vi "mod_Doppler Filter Taps.vi"(0 "doppler spread (hz)":dbl=0.001 format="%#_6p", 5 "fs":dbl=10.0, 7 "doppler filter length":i32=1000, 11 "error in (no error)":errorcluster, 13 "reset? (T)":bool=TRUE) -> (4 "doppler filter taps":dbl[](array[numeric]), 6 "doppler spectrum":dbl[](array[numeric]), 15 "error out":errorcluster)   [LabVIEW 2020, in "niDMT.lvlib"]
doc: "Design of a Doppler filter with U-shaped power spectral density in frequency domain.\n\n\n Inputs:\n 1) Doppler frequency (Hz) \n - range : double precision\n 2) sampling frequency : the sampling frequency of the input\n 3) number of frequency samples within Doppler frequency: the number of samples within the Doppler frequency in frequency domain, which mainly decides the resolution of the filter\n\n Outputs:\n 1) Doppler filter : the Doppler filter coefficient in frequency domain"
uses:
  <vilib>/addons/Modulation/niDMT.lvlib
  <vilib>/Analysis/2dsp.llb/Inverse Real FFT.vi
  <vilib>/Analysis/NI_AALPro.lvlib
panel:
  out "doppler spectrum":cluster{dbl, dbl, dbl[]}(graph)={-0.005, 0.0001, [0.0, 0.0, 0.0, 0.0, 0.0, 0.0, 0.0, 0.0, 0.0, 0.0, 0.0, 0.0, 0.0, 0.0, 0.0, 0.0, 0.0, 0.0, 0.0, 0.0, 0.0, 0.0, 0.0, 0.0, 0.0, 0.0, 0.0, 0.0, 0.0, 0.0, 0.0, 0.0, 0.0, 0.0, 0.0, 0.0, 0.0, 0.0, 0.0, 0.0, 3.3096517068365974, 2.8209479177387817, 2.5857000817159306, 2.4430125595146, 2.3480393851504964, 2.2824478932324883, 2.2372285100045572, 2.2075110436214076, 2.19059400363999, 2.1850968611841584, 2.1850968611841584, 2.19059400363999, 2.2075110436214076, 2.2372285100045572, 2.2824478932324883, 2.3480393851504964, 2.4430125595146, 2.5857000817159306, 2.8209479177387817, 3.3096517068365974, 0.0, 0.0, 0.0, 0.0, 0.0, 0.0, 0.0, 0.0, 0.0, 0.0, 0.0, 0.0, 0.0, 0.0, 0.0, 0.0, 0.0, 0.0, 0.0, 0.0, 0.0, 0.0, 0.0, 0.0, 0.0, 0.0, 0.0, 0.0, 0.0, 0.0, 0.0, 0.0, 0.0, 0.0, 0.0, 0.0, 0.0, 0.0, 0.0, 0.0]}
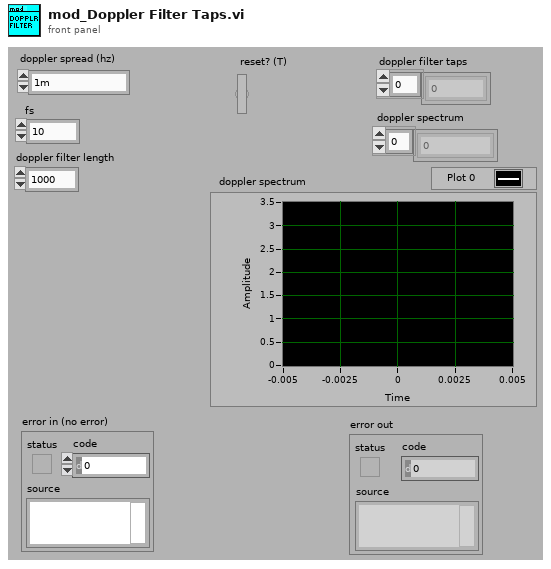
[diagram p1: front panel]
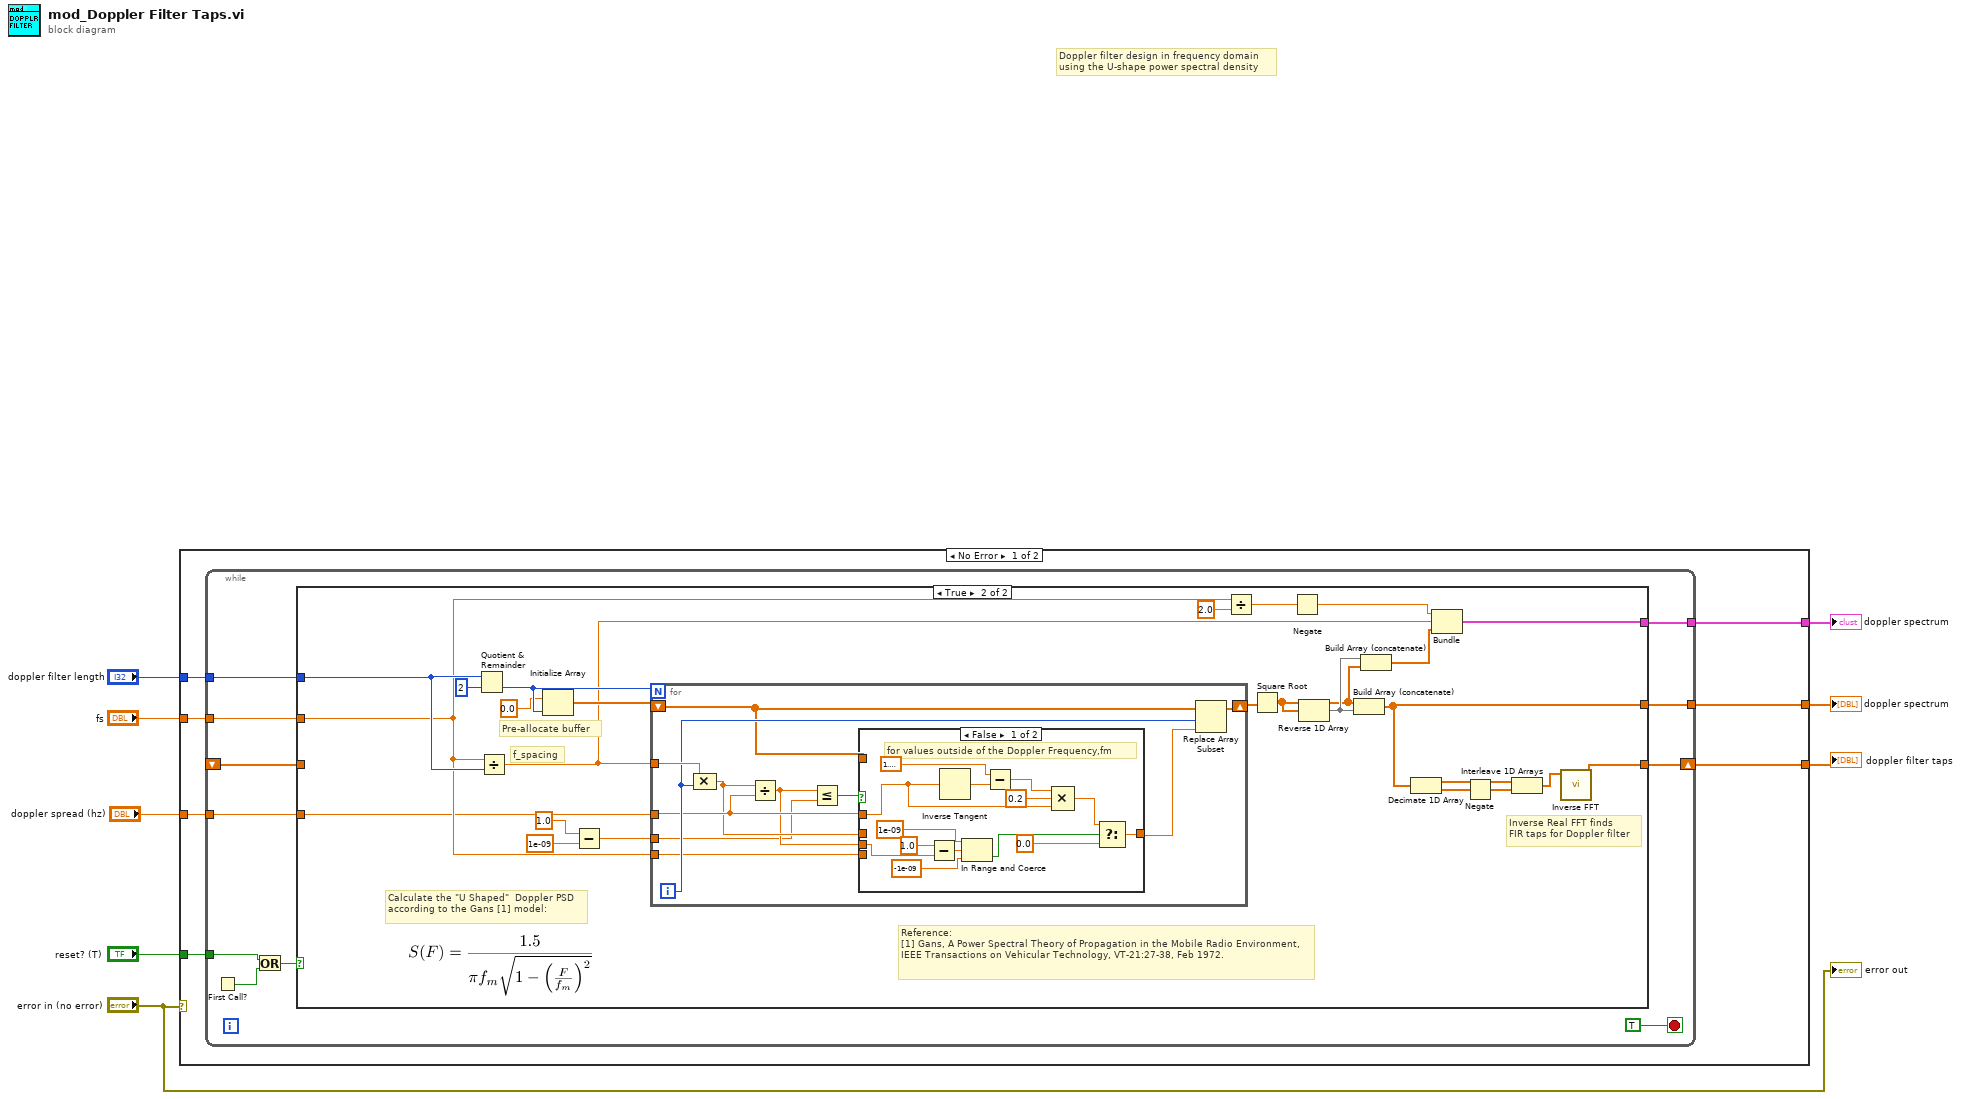
[diagram p0: block diagram]
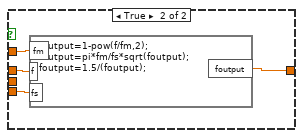
[diagram p3: hidden frame]
diagram:
  # "Doppler filter design in frequency domain\nusing the U-shape power spectral density"
  n1 = case shown="No Error" "error in (no error)" {
    tunnel: "doppler filter length" -> [w15 _]
    tunnel: "fs" -> [w14 _]
    tunnel: "doppler spread (hz)" -> [w13 _]
    tunnel: "reset? (T)" -> [w12 _]
    tunnel: [w11 _] -> w3
    tunnel: [w10 _] -> w2
    tunnel: [w9 _] -> w1
    frame No Error {
      n2 = while {
        shift-right: [w25] -> w11
        shift-left: _ -> [w22]
        tunnel: w15 -> [w21]
        tunnel: w14 -> [w20]
        tunnel: w13 -> [w19]
        tunnel: w12 -> [w18]
        tunnel: [w17] -> w10
        tunnel: [w16] -> w9
        stop <- TRUE stop-if-true
        n3 = First Call?() -> (First Call?: T/F=w24:bool)
        n4 = Or(x=w18, y=w24) -> (x .or. y?=w23:bool)
        n5 = case shown="True" w23 {
          tunnel: [w27 w37] -> w25
          tunnel: w22 -> [w27 _]
          tunnel: w21 -> [_ w32]
          tunnel: w20 -> [_ w31]
          tunnel: w19 -> [_ w30]
          tunnel: [_ w29] -> w17
          tunnel: [_ w28] -> w16
          frame False {
          }
          frame True {
            # "f_spacing"
            # "Inverse Real FFT finds\nFIR taps for Doppler filter"
            # "Pre-allocate buffer"
            # "Reference:\n[1] Gans, A Power Spectral Theory of Propagation in the Mobile Radio Environment, IEEE Transactions on Vehicular Technology, VT-21:27-38, Feb 1972."
            # "Calculate the \"U Shaped\"  Doppler PSD according to the Gans [1] model:"
            n6 = Quotient & Remainder(x=w32, y=2) -> (floor(x/y)=w51:i32)  [unwired: 1 out]
            n7 = Divide(x=w31, y=w32) -> (x/y=w36:dbl)
            n8 = Initialize Array(0.0 ("element"), w51) -> (w49:dbl[])
            n9 = Subtract(x=1.0, y=1e-09) -> (x-y=w33:dbl)
            n10 = for {
              N: w51 -> [_]
              tunnel: w36 -> [w63]
              shift-right: [w62] -> w48
              shift-left: w49 -> [w59]
              tunnel: w30 -> [w57]
              tunnel: w31 -> [w58]
              tunnel: w33 -> [w53]
              i -> [w60]
              n11 = Compound Arithmetic op=MULTIPLY(w63, w60) -> (w55:dbl)
              n12 = Divide(x=w55, y=w57) -> (x/y=w54:dbl)
              n13 = Less Or Equal?(x=w54, y=w53) -> (x <= y?=w56:bool)
              n14 = case shown="False" w56 {
                tunnel: w55 -> [_ w80]
                tunnel: [w76 w81] -> w61
                tunnel: w57 -> [w71 w79]
                tunnel: w59 -> [_ _]
                tunnel: w58 -> [_ w78]
                tunnel: w54 -> [w68 _]
                frame False {
                  # "for values outside of the Doppler Frequency,fm"
                  n15 = Subtract(x=1.0, y=w68) -> (x-y=w67:dbl)
                  n16 = Inverse Tangent(1:w71) -> (0:w73:dbl)
                  n17 = In Range and Coerce(upper limit=1e-09 ("x"), x=w67, lower limit=-1e-09 ("x")) -> (In Range?=w75:bool)  [unwired: 1 out]
                  n18 = Subtract(x=1.5707963267948966, y=w73) -> (x-y=w72:dbl)
                  n19 = Compound Arithmetic op=MULTIPLY(w72, 0.2 ("value"), w71) -> (w69:dbl)
                  n20 = Select(t=w69, s=w75, f=0.0) -> (s? t:f=w76:dbl)
                }
                frame True {
                  n21 = formula code="foutput=1-pow(f/fm,2);\nfoutput=pi*fm/fs*sqrt(foutput);\nfoutput=1.5/(foutput);"("f"=w80, "fm"=w79, "fs"=w78) -> ("foutput"=w81:dbl)
                }
              }
              n22 = Replace Array Subset(array=w59, new element=w61, index=w60) -> (w62:dbl[])
            }
            n23 = Divide(x=w31, y=2.0) -> (x/y=w44:dbl)
            n24 = Square Root(x=w48) -> (sqrt(x)=w46:dbl[])
            n25 = Negate(x=w44) -> (-x=w43:dbl)
            n26 = Reverse 1D Array(array=w46) -> (reversed array=w47:dbl[])
            n27 = Build Array (concatenate)(w46, w47) -> (w28:dbl[])
            n28 = Build Array (concatenate)(w47, w46) -> (w42:dbl[])
            n29 = Decimate 1D Array(w28) -> (w39:dbl[], w38:dbl[])
            n30 = Bundle(w43, w36, w42) -> (w29:cluster{dbl, dbl, dbl[]})  [unwired: 1 out]
            n31 = Negate(x=w38) -> (-x=w40:dbl[])
            n32 = Interleave 1D Arrays(w39, w40) -> (w41:dbl[])
            n33 = call-poly <vilib>:"Inverse FFT.vi"("FFT {X}"=w41) -> ("X"=w37:dbl[])  [unwired: 1 in, 9 out]
          }
        }
      }
    }
    frame Error {
    }
  }
  "doppler filter taps" <- w3
  "doppler spectrum" <- w2
  "doppler spectrum" <- w1
  "error out" <- "error in (no error)"
